vi "VI Server_Get TabControl Cluster From Refference w Merging.vi"(8 "error in":errorcluster, 9 "Tab.Control Reference":refnum<vi>, 11 "VI Server Cluster":T1) -> (0 "error out":errorcluster, 2 "VI Server Cluster.OUT":T1={"Labels"=["Label", "Size", "Font", "Heght", "Width", "Ledding Denominator", "Ledding Nominator", "Label Number", "Microstep Resolution", "X", "Y", "Z", "Italic?", "Underlined?"], "Refs"=[], "VI Ref"=refnum} caption="VI Server Cluster.Out")   [LabVIEW 2020, in "VI Server Toolkit LV2013.lvlib"]
doc: "Retrieves control labels and references of a tab control (reference input) and merges it into VI server Cluster."
uses:
  VI Server Toolkit LV2013.lvlib
  VI Server_TypeDefs/VI Server_RefsCluster.ctl
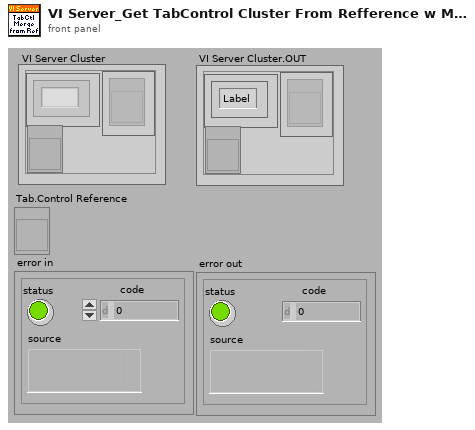
[diagram p1: front panel]
types:
  T1 = typedef "VI Server_RefsCluster.ctl" = cluster{"Labels":string[], "Refs":refnum<vi>[], "VI Ref":refnum<vi>}
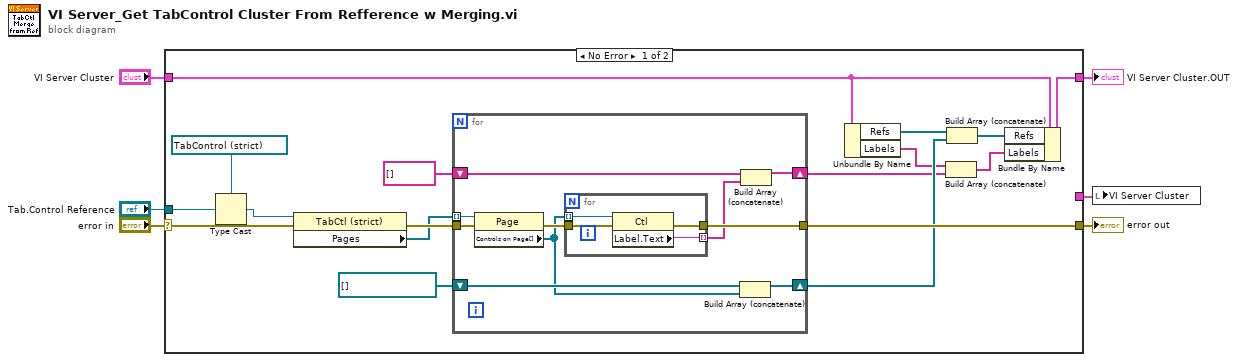
[diagram p0: block diagram]
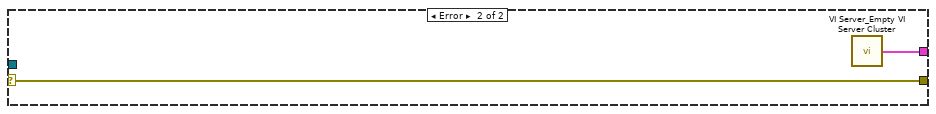
[diagram p2: hidden frame]
diagram:
  n1 = case shown="No Error" "error in" {
    selector: "error in" -> [w18 w39]
    tunnel: "VI Server Cluster" -> [w12 _]
    tunnel: [w23 w39] -> w5
    tunnel: "Tab.Control Reference" -> [w17 _]
    tunnel: [w7 _] -> w2
    tunnel: [_ w38] -> w1
    frame No Error {
      n2 = Type Cast(type=refnum<vi> refnum ("Tab Control Ref"), x=w17) -> (*(type *) &x=w16:refnum<vi>)
      n3 = property class="TabCtl (strict)"(reference=w16, error in=w18) -> (error out=w22:errorcluster, "Pages"=w21:refnum<vi>[])  [unwired: 1 out]
      n4 = for {
        tunnel: w22 -> [w32]
        tunnel: [w30] -> w23
        tunnel: w21 -> [w33] mode=indexing
        shift-right: [w27] -> w9
        shift-left: string[] [] -> [w29]
        shift-right: [w25] -> w13
        shift-left: refnum<vi>[] [] ("Controls on Page[]") -> [w26]
        n5 = property class="Page"(reference=w33, error in=w32) -> (error out=w31:errorcluster, "Controls on Page[]"=w24:refnum<vi>[])  [unwired: 1 out]
        n6 = for {
          tunnel: w31 -> [w37]
          tunnel: w24 -> [w36] mode=indexing
          tunnel: [w35] -> w30
          tunnel: [w34] -> w28 mode=indexing
          n7 = property class="Ctl"(reference=w36, error in=w37) -> (error out=w35:errorcluster, "Label.Text"=w34:string)  [unwired: 1 out]
        }
        n8 = Build Array (concatenate)(w26, w24) -> (w25:refnum<vi>[])
        n9 = Build Array (concatenate)(w29, w28) -> (w27:string[])
      }
      n10 = Unbundle By Name(w12) -> ("Refs"=w14:refnum<vi>[], "Labels"=w10:string[])
      n11 = Build Array (concatenate)(w10, w9) -> (w8:string[])
      n12 = Build Array (concatenate)(w14, w13) -> (w11:refnum<vi>[])
      n13 = Bundle By Name(cluster=w12, "Refs"=w11, "Labels"=w8) -> (w7:T1)
    }
    frame Error {
      n14 = call "VI Server_Empty VI Server Cluster.vi"() -> ("VI Server Cluster"=w38:T1)  [unwired: 7 in]
    }
  }
  "error out" <- w5
  "VI Server Cluster.OUT" <- w2
  n15 = local write "VI Server Cluster"(w1) -> ()
